vi "Delete State Storage.vi"(8 "error in (no error)":errorcluster, 10 "Storage Location (1: 1)":i32(ring)=1 items=["0", "1", "2", "3", "4"], 11 "VISA resource name":refnum<visa-resource-name>) -> (0 "error out":errorcluster, 3 "VISA resource name out":refnum<visa-resource-name>)   [LabVIEW 2020, in "Agilent 3352X Series.lvlib"]
doc: "Deletes the contents of the specified storage location.\n\n<b>Note</b>:\nIf you have named a storage location deleting the contents of a storage location will reset the associated name to its factory default (\"AUTO RECALL\", \"STATE_1\", \"STATE_2\", \"STATE_3\", or \"STATE_4\")."
uses:
  Agilent 3352X Series.lvlib
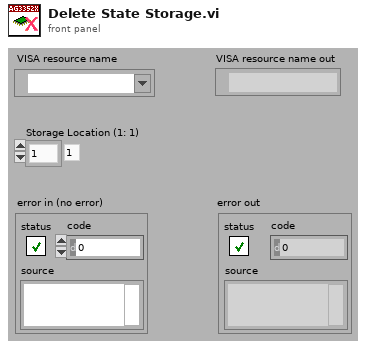
[diagram p1: front panel]
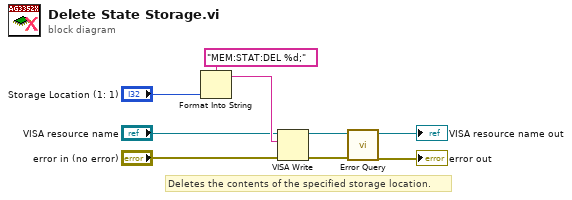
[diagram p0: block diagram]
diagram:
  # "Deletes the contents of the specified storage location."
  n1 = Format Into String(format string="MEM:STAT:DEL %d;", "Storage Location (1: 1)") -> (resulting string=w7:string)  [unwired: 2 in, 1 out]
  n2 = VISA Write(VISA resource name="VISA resource name", write buffer=w7, error in (no error)="error in (no error)") -> (VISA resource name out=w4:refnum<visa-resource-name>, error out=w3:errorcluster)  [unwired: 1 out]
  n3 = call "Error Query.vi"("error in (no error)"=w3, "VISA resource name"=w4) -> ("error out"=→"error out":errorcluster, "VISA resource name out"=→"VISA resource name out":refnum<visa-resource-name>)  [unwired: 8 out]
